vi "Elevator Auto Set State.vi"(8 "error in (no error)":errorcluster, 10 "New State":T1=enum."Tote 1") -> (0 "error out":errorcluster)   [LabVIEW 2014]
uses:
  Elevator States.ctl
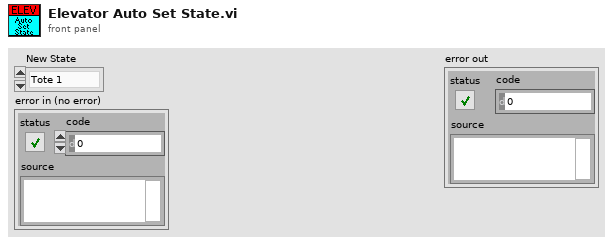
[diagram p1: front panel]
types:
  T1 = typedef "Elevator States.ctl" = enum16{"Ground", "Tote 1", "Tote 2", "Tote 3", "Tote 4", "Tote 5", "Tote 6"}
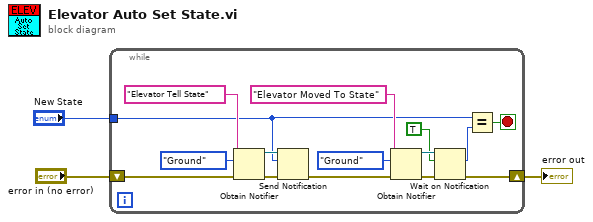
[diagram p0: block diagram]
diagram:
  n1 = while {
    tunnel: "New State" -> [w12]
    shift-right: [w7] -> w1
    shift-left: "error in (no error)" -> [w8]
    stop <- w6 stop-if-true
    n2 = Obtain Notifier(name (unnamed)="Elevator Tell State", notification data type=Elevator_States."Ground" ("Output State"), error in (no error)=w8) -> (notifier out=w16:refnum<notifier>, error out=w11:errorcluster)  [unwired: 1 in, 1 out]
    n3 = Send Notification(notification=w12, notifier=w16, error in (no error)=w11) -> (error out=w10:errorcluster)  [unwired: 1 out]
    n4 = Obtain Notifier(name (unnamed)="Elevator Moved To State", notification data type=Elevator_States."Ground" ("Output State"), error in (no error)=w10) -> (notifier out=w15:refnum<notifier>, error out=w9:errorcluster)  [unwired: 1 in, 1 out]
    n5 = Wait on Notification(notifier=w15, ignore previous (F)=TRUE, error in (no error)=w9) -> (notification=w13:T1, error out=w7:errorcluster)  [unwired: 1 in, 2 out]
    n6 = Equal?(x=w12, y=w13) -> (x = y?=w6:bool)
  }
  "error out" <- w1
